vi "Init.vi"(8 "error in (no error)":errorcluster, 11 "UI Actor in":refnum<class "UI Actor.lvclass">) -> (0 "error out":errorcluster, 3 "UI Actor out":refnum<class "UI Actor.lvclass">)   [LabVIEW 2019, in "UI Actor.lvlib" / "UI Actor.lvclass"]
uses:
  UI Actor.lvclass
  C:/Program Files (x86)/National Instruments/LabVIEW 2019/vi.lib/ActorFramework/Actor/Actor.lvclass
  MENSAJES/MENSAJES.lvclass
  UI Actor.lvclass/UI Actor.ctl
  MXN Actor/MXN Actor.lvclass
  MXN Actor/MXN Actor.lvclass/MXN Actor.ctl
  USD Actor/USD Actor.lvclass
  USD Actor/USD Actor.lvclass/USD Actor.ctl
  REFRESCOS Y PAPAS ACTOR/REFRESCOS Y PAPAS ACTOR.lvclass
  REFRESCOS Y PAPAS ACTOR/REFRESCOS Y PAPAS ACTOR.lvclass/REFRESCOS Y PAPAS ACTOR.ctl
  CAFE ACTOR/CAFE ACTOR.lvclass
  CAFE ACTOR/CAFE ACTOR.lvclass/CAFE ACTOR.ctl
  MENSAJES/MENSAJES.lvclass/MENSAJES.ctl
  Read Mensajes.vi
  Read Monedas.vi
  Read Sub Panel Monedas.vi
  Read Productos.vi
  Read Sub Panel Productos.vi
  Read Sub Panel Msg.vi
  <vilib>/ActorFramework/Actor/Actor.lvclass
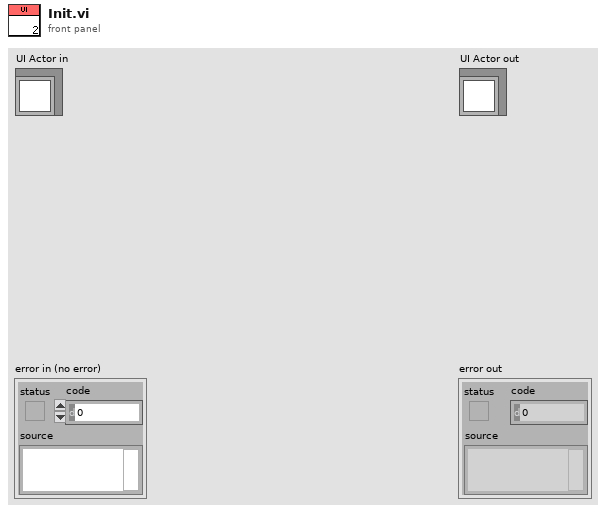
[diagram p1: front panel]
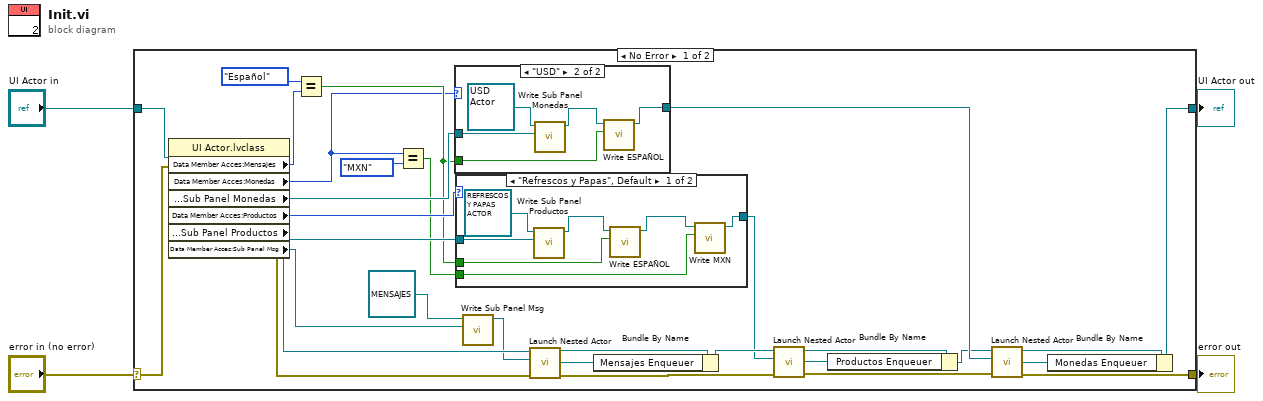
[diagram p0: block diagram]
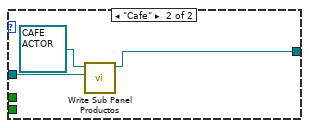
[diagram p2: hidden frame]
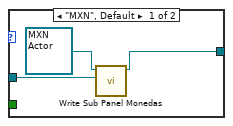
[diagram p3: hidden frame]
diagram:
  n1 = case shown="No Error" "error in (no error)" {
    selector: "error in (no error)" -> [w33 w54]
    tunnel: [w34 w54] -> w3
    tunnel: [w29 w53] -> w1
    tunnel: "UI Actor in" -> [w32 w53]
    frame No Error {
      n2 = property class="UI Actor.lvclass"(reference=w32, error in=w33) -> (reference out=w18:refnum<class "UI Actor.lvclass">, error out=w17:errorcluster, "Data Member Acces:Mensajes"=w10:enum16{"Ingles", "Español"}, "Data Member Acces:Monedas"=w7:enum16{"MXN", "USD"}, "Data Member Acces:Sub Panel Monedas"=w27:refnum<vi>, "Data Member Acces:Productos"=w26:enum16{"Refrescos y Papas", "Cafe"}, "Data Member Acces:Sub Panel Productos"=w25:refnum<vi>, "Data Member Acces:Sub Panel Msg"=w11:refnum<vi>)
      n3 = Equal?(x=enum16{"Ingles", "Español"}."Español" ("t"), y=w10) -> (x = y?=w8:bool)
      n4 = Equal?(x=w7, y=enum16{"MXN", "USD"}."MXN") -> (x = y?=w5:bool)
      n5 = case shown="\"USD\"" w7 {
        tunnel: [w45 w50] -> w30
        tunnel: w27 -> [w46 w52]
        tunnel: w8 -> [_ w48]
        frame "MXN", Default {
          n6 = call "Write Sub Panel Monedas.vi"("Sub Panel Monedas"=w46, "MXN Actor in"=refnum<class "MXN Actor.lvclass"> refnum ("MXN Actor.lvlib:MXN Actor.lvclass")) -> ("MXN Actor out"=w45:refnum<class "MXN Actor.lvclass">)  [unwired: 8 in, 1 out]
        }
        frame "USD" {
          n7 = call "Write Sub Panel Monedas.vi"("Sub Panel Monedas"=w52, "USD Actor in"=refnum<class "USD Actor.lvclass"> refnum ("USD Actor.lvlib:USD Actor.lvclass")) -> ("USD Actor out"=w49:refnum<class "USD Actor.lvclass">)  [unwired: 8 in, 1 out]
          n8 = call "Write ESPAÑOL.vi"("ESPAÑOL"=w48, "USD Actor in"=w49) -> ("USD Actor out"=w50:refnum<class "USD Actor.lvclass">)  [unwired: 8 in, 1 out]
        }
      }
      n9 = case shown="\"Refrescos y Papas\", Default" w26 {
        tunnel: w25 -> [w40 w44]
        tunnel: [w37 w42] -> w12
        tunnel: w8 -> [w36 _]
        tunnel: w5 -> [w35 _]
        frame "Refrescos y Papas", Default {
          n10 = call "Write Sub Panel Productos.vi"("Sub Panel Productos"=w40, "REFRESCOS Y PAPAS ACTOR in"=refnum<class "REFRESCOS Y PAPAS ACTOR.lvclass"> refnum ("REFRESCOS Y PAPAS ACTOR.lvlib:REFRESCOS Y PAPAS ACTOR.lvclass")) -> ("REFRESCOS Y PAPAS ACTOR out"=w39:refnum<class "REFRESCOS Y PAPAS ACTOR.lvclass">)  [unwired: 8 in, 1 out]
          n11 = call "Write ESPAÑOL.vi"("ESPAÑOL"=w36, "REFRESCOS Y PAPAS ACTOR in"=w39) -> ("REFRESCOS Y PAPAS ACTOR out"=w38:refnum<class "REFRESCOS Y PAPAS ACTOR.lvclass">)  [unwired: 8 in, 1 out]
          n12 = call "Write MXN.vi"("MXN"=w35, "REFRESCOS Y PAPAS ACTOR in"=w38) -> ("REFRESCOS Y PAPAS ACTOR out"=w37:refnum<class "REFRESCOS Y PAPAS ACTOR.lvclass">)  [unwired: 8 in, 1 out]
        }
        frame "Cafe" {
          n13 = call "Write Sub Panel Productos.vi"("Sub Panel Productos"=w44, "CAFE ACTOR in"=refnum<class "CAFE ACTOR.lvclass"> refnum ("CAFE ACTOR.lvlib:CAFE ACTOR.lvclass")) -> ("CAFE ACTOR out"=w42:refnum<class "CAFE ACTOR.lvclass">)  [unwired: 8 in, 1 out]
        }
      }
      n14 = call "Write Sub Panel Msg.vi"("Sub Panel Msg"=w11, "MENSAJES in"=refnum<class "MENSAJES.lvclass"> refnum ("MENSAJES.lvlib:MENSAJES.lvclass")) -> ("MENSAJES out"=w15:refnum<class "MENSAJES.lvclass">)  [unwired: 8 in, 1 out]
      n15 = call <vilib>:"Launch Nested Actor.vi"("error in (no error)"=w17, "Nested Actor"=w15, "Caller Actor in"=w18) -> ("error out"=w16:errorcluster, "Nested Actor's Enqueuer"=w13:refnum<class "Message Enqueuer.lvclass">, "Caller Actor out"=w19:refnum<class "UI Actor.lvclass">)  [unwired: 6 in]
      n16 = Bundle By Name(cluster=w19, "Mensajes Enqueuer"=w13) -> (w14:refnum<class "UI Actor.lvclass">)
      n17 = call <vilib>:"Launch Nested Actor.vi"("error in (no error)"=w16, "Nested Actor"=w12, "Caller Actor in"=w14) -> ("error out"=w22:errorcluster, "Nested Actor's Enqueuer"=w24:refnum<class "Message Enqueuer.lvclass">, "Caller Actor out"=w23:refnum<class "UI Actor.lvclass">)  [unwired: 6 in]
      n18 = Bundle By Name(cluster=w23, "Productos Enqueuer"=w24) -> (w21:refnum<class "UI Actor.lvclass">)
      n19 = call <vilib>:"Launch Nested Actor.vi"("error in (no error)"=w22, "Nested Actor"=w30, "Caller Actor in"=w21) -> ("error out"=w34:errorcluster, "Nested Actor's Enqueuer"=w28:refnum<class "Message Enqueuer.lvclass">, "Caller Actor out"=w31:refnum<class "UI Actor.lvclass">)  [unwired: 6 in]
      n20 = Bundle By Name(cluster=w31, "Monedas Enqueuer"=w28) -> (w29:refnum<class "UI Actor.lvclass">)
    }
    frame Error {
    }
  }
  "error out" <- w3
  "UI Actor out" <- w1
